vi "BoxSimArm.vi"() -> ()   [LabVIEW 2023]
uses:
  <vilib>/Rock Robotics/WPI/ThirdParty/JAS_Junk/TrajLib/Enum/DCMOTOR_TYPES_ENUM.ctl
  <vilib>/Rock Robotics/WPI/ThirdParty/JAS_Junk/TrajLib/VI/Util_GetTime_U32.vi
  <vilib>/Rock Robotics/WPI/ThirdParty/JAS_Junk/TrajLib/VI/numCmd_ObtainQueue_OneDbl.vi
  <vilib>/Rock Robotics/WPI/ThirdParty/JAS_Junk/TrajLib/SlewRateLimiter_New.vi
  <vilib>/Rock Robotics/WPI/ThirdParty/JAS_Junk/TrajLib/SlewRateLimiter_Reset.vi
  <vilib>/Rock Robotics/WPI/ThirdParty/JAS_Junk/TrajLib/SlewRateLimiter_Calculate.vi
  <vilib>/Rock Robotics/WPI/ThirdParty/JAS_Junk/TrajLib/SlewRateLimiter_SetRate.vi
  <vilib>/Rock Robotics/WPI/ThirdParty/JAS_Junk/TrajLib/LinearFilter_ResetToValue.vi
  <vilib>/Rock Robotics/WPI/ThirdParty/JAS_Junk/TrajLib/LinearFilter_Calculate.vi
  <vilib>/Rock Robotics/WPI/ThirdParty/JAS_Junk/TrajLib/BatterySim_CalculateLoadedBatteryVoltage.vi
  <vilib>/Rock Robotics/WPI/ThirdParty/JAS_Junk/TrajLib/VI/Util_GetTime_U64.vi
  <vilib>/Rock Robotics/WPI/ThirdParty/JAS_Junk/TrajLib/LinearFilter_MovingAverage.vi
  <vilib>/Rock Robotics/WPI/ThirdParty/JAS_Junk/TrajLib/LinearFilter_LowPassBW1.vi
  <vilib>/Rock Robotics/WPI/ThirdParty/JAS_Junk/TrajLib/LinearFilter_LowPassBW2.vi
  <vilib>/Rock Robotics/WPI/ThirdParty/JAS_Junk/TrajLib/LinearFilter_HighPassBW1.vi
  <vilib>/Rock Robotics/WPI/ThirdParty/JAS_Junk/TrajLib/LinearFilter_HighPassBW2.vi
  <vilib>/Rock Robotics/WPI/ThirdParty/JAS_Junk/TrajLib/Trajectory_Library.lvlib
panel:
  out "Motor Current Filt":dbl
  out "Gravity Comp Output":dbl
  out "Motor Current":dbl
  out "Rev / Lo Lim":bool
  out "Fwd / Hi Lim":bool
  out "Arm Demand Deg":dbl
  out "Battery Voltage":dbl format="%10.1f"
  out "Shooter Control":T1(graph)
  out "Position DEG":dbl format="%13.1f"
  out "AtSetpoint":bool
  in  "Pos Dmd DEG":dbl=90.0 min=-20.0 max=150.0 step=5.0
  out "Motor Dmd (CO)":dbl format="%10.3f"
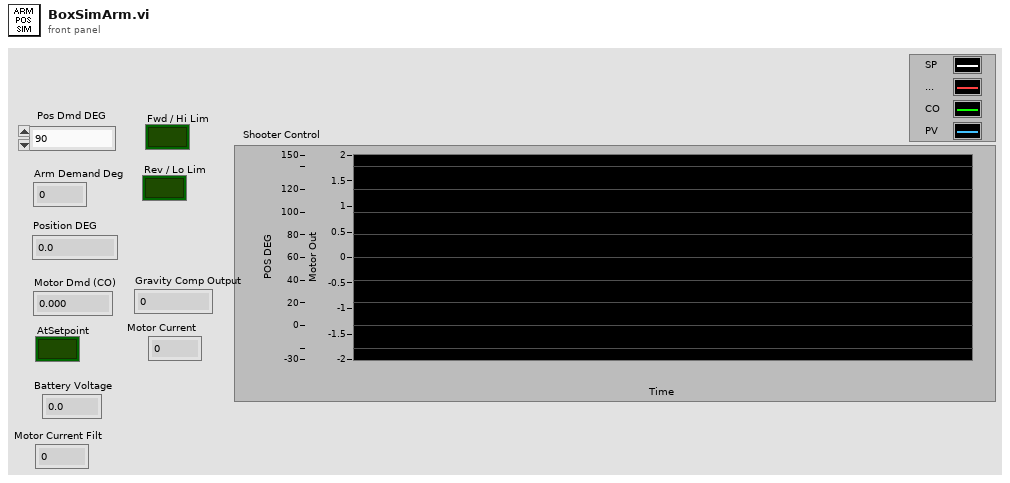
[diagram p1: front panel]
types:
  T1 = cluster{"Setpoint":dbl, "FeedForward":dbl, "CO-ControlOutput":dbl, "Velocity_RPM":dbl}
  T2 = enum16{"Moving Average", "Low Pass 1st Order Butterworth", "Low Pass 2nd Order Butterworth", "High Pass 1st Order Butterworth", "High Pass 2nd Order Butterworth"}
  T3 = typedef "Trajectory_Library.lvlib/DCMOTOR_TYPES_ENUM.ctl" = enum16{"CIM", "AndyMark 9015", "Andy Mark RS 775 125", "Bag", "BaneBots RS 550", "BaneBots RS 775", "Falcon 500", "Mini CIM", "NEO", "NEO 550", "Romi BuiltIn", "Vex 775 Pro", "Snow Blower AM 2235A", "Bosch Seat AM 3493"}
  T4 = typedef "Trajectory_Library.lvlib/LINEAR_SYSTEM_ID_SINGLE_JOINT_ARM_MODEL.ctl" = cluster{"DCMOTOR_TYPES":T3, "Num Motors":i32, "ArmLength_M":dbl, "massKg":dbl, "Gearing":dbl, "MOI kgm2":dbl, "Estimate MOI":bool}
  T5 = typedef "Trajectory_Library.lvlib/SINGLE_JOINT_ARM_SIM_SIMULATION_PARAMS.ctl" = cluster{"MinAngle_Rad":dbl, "MaxAngle_Rad":dbl, "Measurment StdDev":dbl, "SimulateGravity":bool}
  T6 = cluster{"Pos Dmd DEG":dbl, "Arm Demand Deg":dbl, "Motor Output":dbl, "Degrees":dbl}
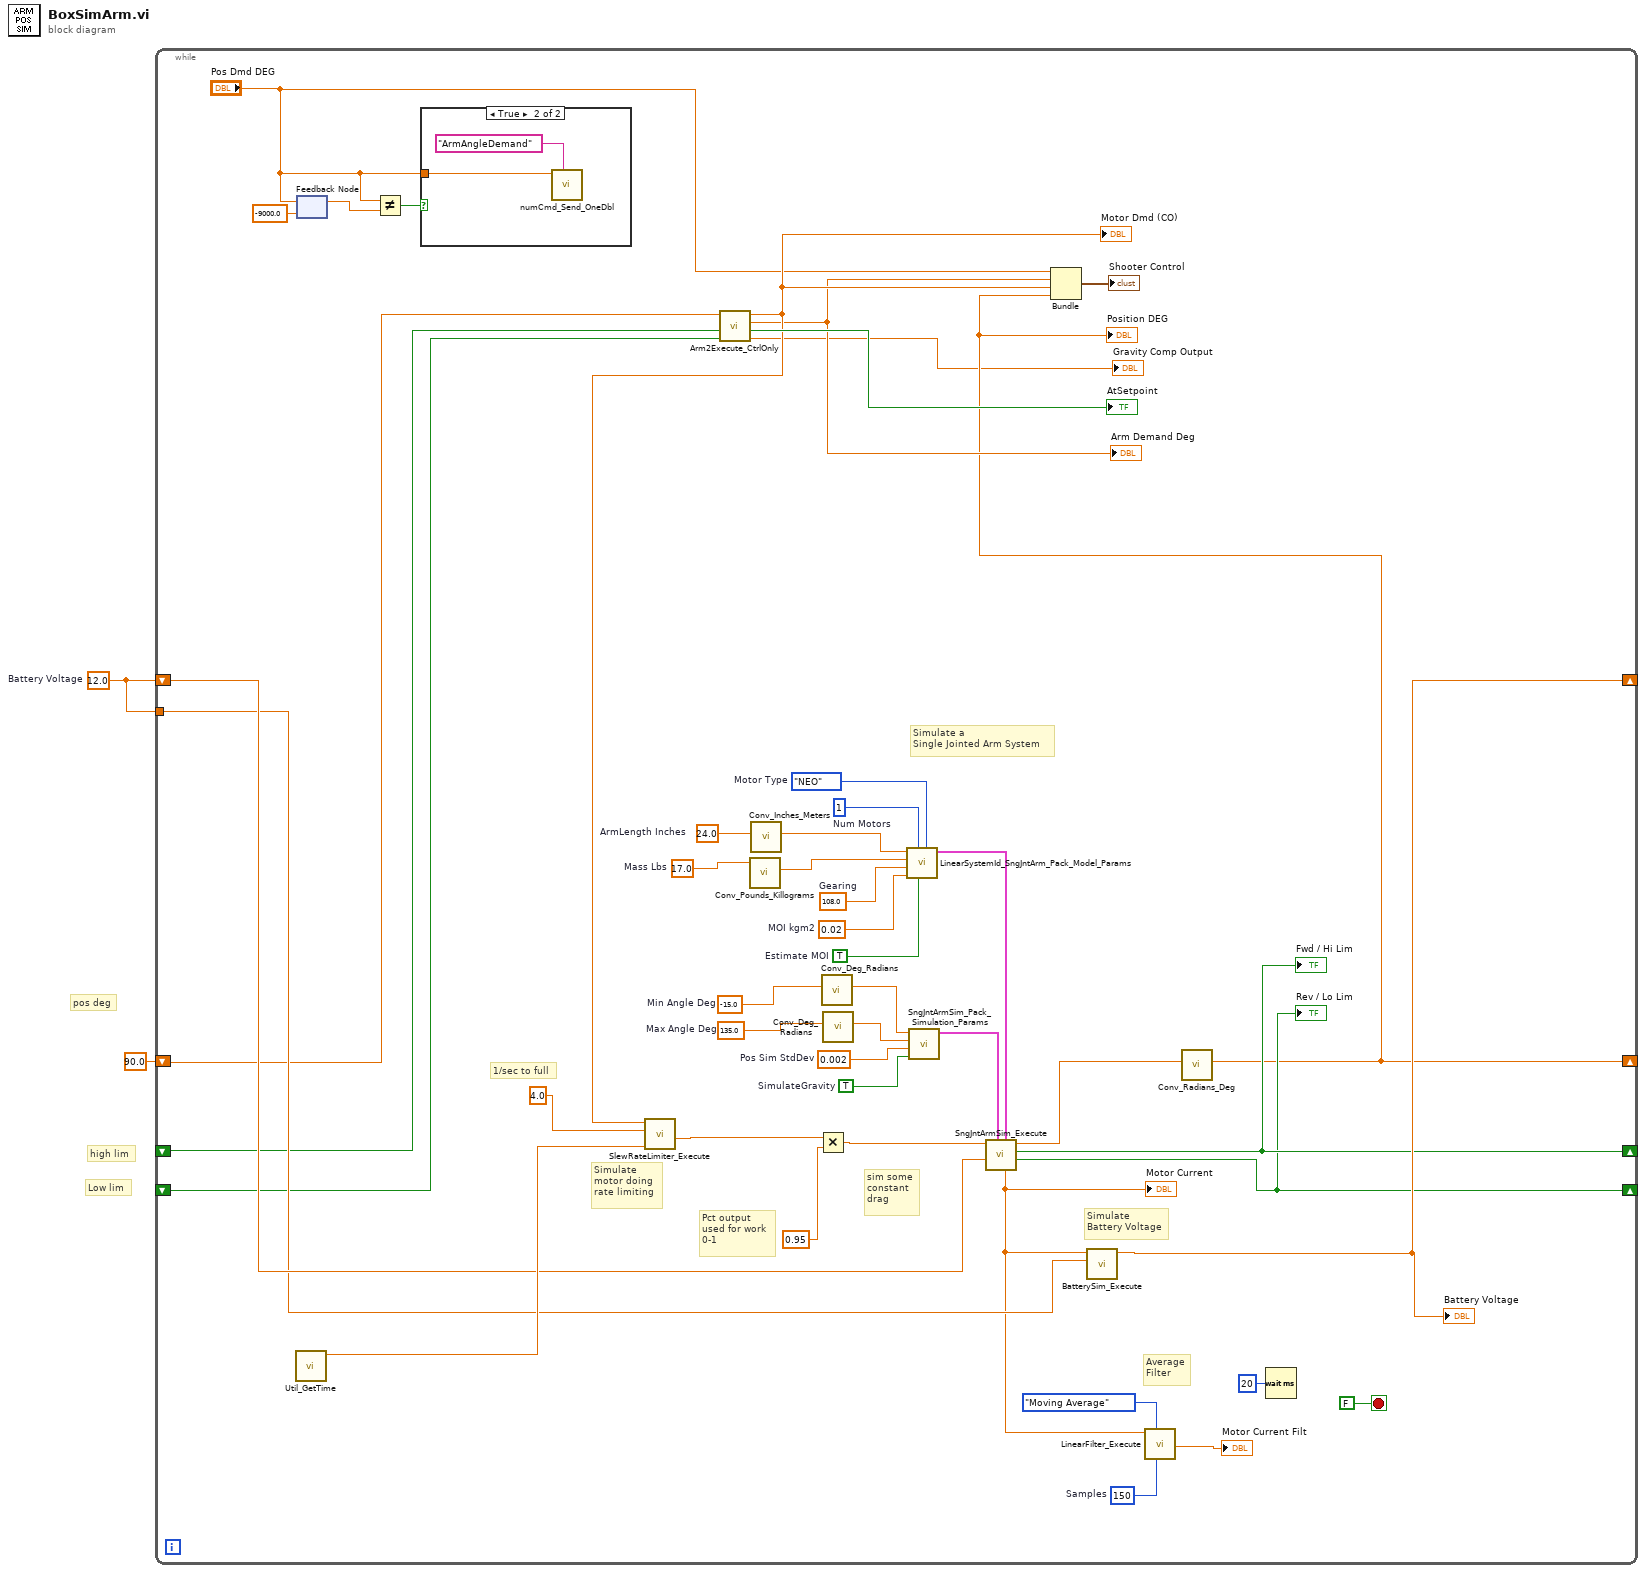
[diagram p0: block diagram]
diagram:
  w2 = 12.0  # Battery Voltage
  # "pos deg"
  # "Low lim"
  # "high lim"
  n1 = while {
    shift-right: [w21] -> _
    shift-left: w2 -> [w33]
    shift-right: [w9] -> _
    shift-left: 90.0 ("Degrees") -> [w17]
    tunnel: w2 -> [w32]
    shift-right: [w11] -> _
    shift-left: _ -> [w16]
    shift-right: [w10] -> _
    shift-left: _ -> [w15]
    stop <- FALSE stop-if-true
    w6 = 150  # Samples
    w36 = TRUE  # Estimate MOI
    w37 = 0.02  # MOI kgm2
    w31 = -15.0  # Min Angle Deg
    w30 = 135.0  # Max Angle Deg
    w38 = 0.002  # Pos Sim StdDev
    w39 = TRUE  # SimulateGravity
    w25 = 24.0  # ArmLength Inches
    w40 = 108.0  # Gearing
    w26 = 17.0  # Mass Lbs
    w41 = 1  # Num Motors
    w42 = DCMOTOR_TYPES_ENUM."NEO"  # Motor Type
    # "Average\nFilter"
    # "1/sec to full"
    # "Simulate\nBattery Voltage"
    # "Simulate a\nSingle Jointed Arm System"
    # "Pct output\nused for work\n0-1"
    # "Simulate\nmotor doing\nrate limiting"
    # "sim some\nconstant\ndrag"
    n2 = call <vilib>:"Util_GetTime.vi"() -> ("FPGA_Time_Seconds"=w43:dbl)  [unwired: 9 in, 2 out]
    n3 = feedback-in #1("Pos Dmd DEG") -> ()
    n4 = feedback #1(-9000.0 ("Pos Dmd DEG")) -> (w12:dbl)
    n5 = Not Equal?(x="Pos Dmd DEG", y=w12) -> (x != y?=w14:bool)
    n6 = case shown="True" w14 {
      tunnel: "Pos Dmd DEG" -> [_ w50]
      frame False {
      }
      frame True {
        n7 = call <vilib>:"numCmd_Send_OneDbl.vi"("Command Name"="ArmAngleDemand", "Value"=w50) -> ()  [unwired: 9 in, 1 out]
      }
    }
    n8 = call "Arm2Execute_CtrlOnly.vi"("ReverseLimitSwitch"=w15, "ForwardLimitSwitch"=w16, "SensorPos Deg"=w17) -> ("Gravity Comp Output"=→"Gravity Comp Output":dbl, "OnTarget"=→"AtSetpoint":bool, "Arm Demand Deg"=w18:dbl, "Motor Output"=w19:dbl)  [unwired: 5 in]
    "Motor Dmd (CO)" <- w19
    "Arm Demand Deg" <- w18
    n9 = call <vilib>:"SlewRateLimiter_Execute.vi"("Time"=w43, "PositiveRate"=4.0 ("y"), "Input"=w19) -> ("Output"=w46:dbl)  [unwired: 7 in, 1 out]
    n10 = call <vilib>:"Conv_Pounds_Killograms.vi"("Pounds"=w26) -> ("Killograms"=w27:dbl)  [unwired: 10 in]
    n11 = call <vilib>:"Conv_Inches_Meters.vi"("INCH"=w25) -> ("Meters"=w24:dbl)  [unwired: 10 in]
    n12 = Multiply(x=w46, y=0.95) -> (x*y=w23:dbl)
    n13 = call <vilib>:"Conv_Deg_Radians.vi"("Degress"=w31) -> ("Radians"=w29:dbl)  [unwired: 10 in]
    n14 = call <vilib>:"Conv_Deg_Radians.vi"("Degress"=w30) -> ("Radians"=w28:dbl)  [unwired: 10 in]
    n15 = call <vilib>:"LinearSystemId_SngJntArm_Pack_Model_Params.vi"("DCMOTOR_TYPES"=w42, "Estimate MOI"=w36, "Num Motors"=w41, "MOI kgm2"=w37, "Gearing"=w40, "massKg"=w27, "ArmLength_M"=w24) -> ("SngJntArmSim_Model _Params"=w35:T4)  [unwired: 4 in]
    n16 = call <vilib>:"SngJntArmSim_Pack_Simulation_Params.vi"("SimulateGravity"=w39, "Pos Sim StdDev Rad"=w38, "MaxAngle_Rad"=w28, "MinAngle_Rad"=w29) -> ("SngJntArmSim_Simulation _Params"=w34:T5)  [unwired: 7 in]
    n17 = call <vilib>:"SngJntArmSim_Execute.vi"("SngJntArmSim_Model _Params"=w35, "SngJntArmSim_Simulation _Params"=w34, "Battery Volts"=w33, "Motor Dmd"=w23) -> ("AtLowLimit"=w10:bool, "At HIgh LImit"=w11:bool, "ArmAngle_Rad"=w22:dbl, "Motor Current"=w4:dbl)  [unwired: 2 in, 2 out]
    "Fwd / Hi Lim" <- w11
    "Rev / Lo Lim" <- w10
    "Motor Current" <- w4
    n18 = call <vilib>:"BatterySim_Execute.vi"("Nominal Battery Voltage"=w32, "Current"=w4) -> ("Voltage"=w21:dbl)  [unwired: 9 in]
    "Battery Voltage" <- w21
    n19 = call <vilib>:"LinearFilter_Execute.vi"("Samples"=w6, "Filter Type"=T2."Moving Average", "Input"=w4) -> ("Output"=→"Motor Current Filt":dbl)  [unwired: 7 in, 1 out]
    n20 = call <vilib>:"Conv_Radians_Deg.vi"("Radians"=w22) -> ("Degrees"=w9:dbl)  [unwired: 10 in]
    "Position DEG" <- w9
    n21 = Bundle("Pos Dmd DEG"="Pos Dmd DEG", "Arm Demand Deg"=w18, "Motor Output"=w19, "Degrees"=w9) -> (→"Shooter Control":T6)  [unwired: 1 in]
    n22 = Wait (ms)(milliseconds to wait=u32 20) -> ()  [unwired: 1 out]
  }
